vi "Zero-Pole.vi"   [LabVIEW 2020, in "NI_AdvCtrl_continuous linear.lvlib"]
doc: "LabVIEW no longer supports this VI. You can obtain similar functionality by installing the LabVIEW Simulation Module.\n\nCalculates the new output point, where the transfer function and the input point are given. The transfer function is described in gain-zeros-poles notation."
uses:
  <vilib>/addons/control/advanced/NI_AdvCtrl_continuous linear.lvlib
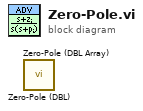
[diagram p0: block diagram]
diagram:
  n1 = call <vilib>:"Zero-Pole (DBL).vi"() -> ()  [unwired: 5 in, 1 out]
  n2 = call <vilib>:"Zero-Pole (DBL Array).vi"() -> ()  [unwired: 5 in, 1 out]
